vi "HandDetector.vi"(6 "Enum":T2, 8 "error in (no error)":errorcluster, 10 "Image":T1, 11 "session in":refnum<k35>) -> (0 "error out":errorcluster, 1 "Landmarkers coords":u32[][](array[numeric]), 2 "OutImage":T1, 3 "session out":refnum<k35>, 4 "HandExist?":bool)   [LabVIEW 2024]
uses:
  #VisionProcessingEnum.ctl
  <vilib>/vision/Image Controls.llb/IMAQ Image.ctl
  <vilib>/Python/Open Venv Python Session.vi
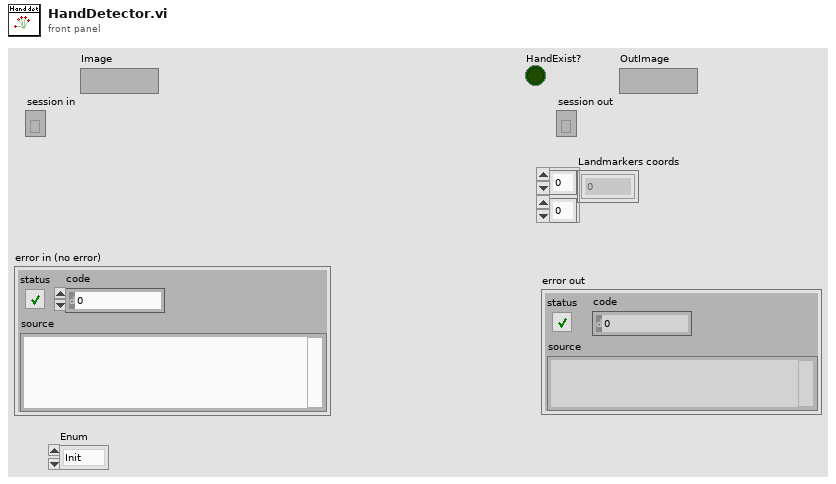
[diagram p1: front panel]
types:
  T1 = typedef "IMAQ Image.ctl" = refnum<image>
  T2 = typedef "#VisionProcessingEnum.ctl" = enum16{"Init", "Processing", "ProcessingVision", "Close"}
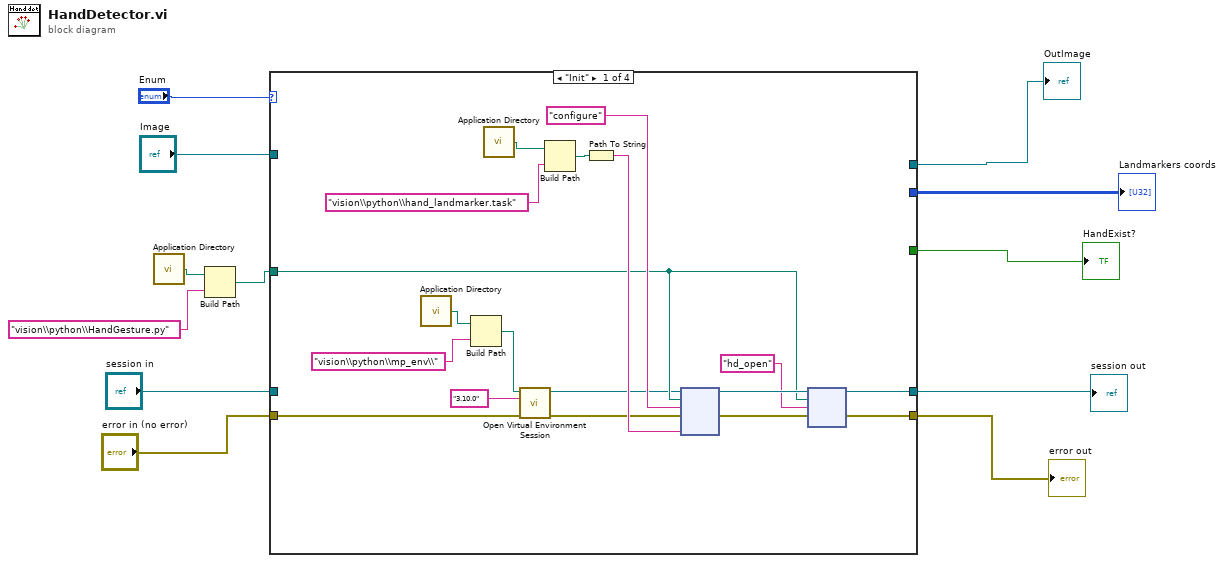
[diagram p0: block diagram]
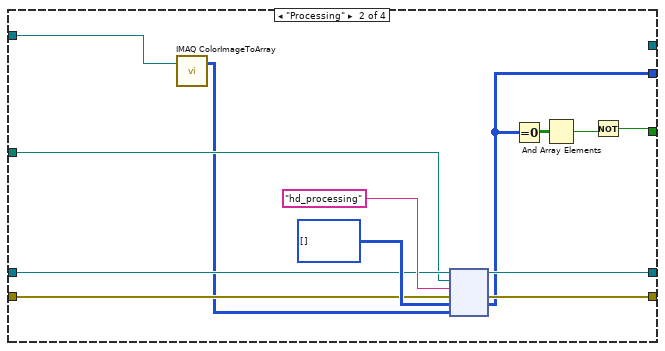
[diagram p2: hidden frame]
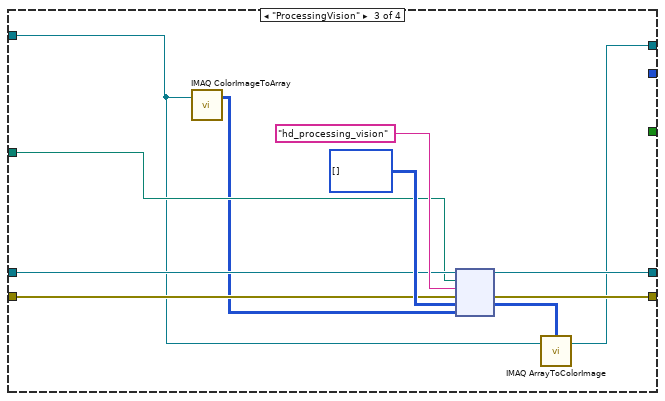
[diagram p3: hidden frame]
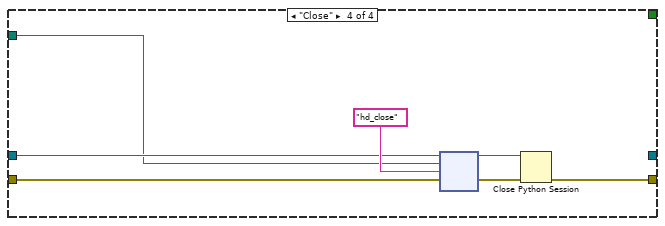
[diagram p4: hidden frame]
diagram:
  n1 = call <vilib>:"Application Directory.vi"() -> ("Application Directory"=w1:path)
  n2 = Build Path(base path=w1, name or relative path="vision\\python\\HandGesture.py" ("function name")) -> (appended path=w6:path)
  n3 = case shown="\"Init\"" "Enum" {
    tunnel: [w23 w40 w52 _] -> w9
    tunnel: [w22 w41 w50 w58] -> w8
    tunnel: "error in (no error)" -> [w13 w38 w49 w57]
    tunnel: "session in" -> [_ w39 w51 w56]
    tunnel: [_ _ w46 _] -> w4
    tunnel: w6 -> [w21 w37 w48 w55]
    tunnel: "Image" -> [_ w35 w44 _]
    tunnel: [_ w34 _ _] -> w3
    tunnel: [_ w31 _ _] -> w2
    frame "Init" {
      n4 = call <vilib>:"Application Directory.vi"() -> ("Application Directory"=w18:path)
      n5 = Build Path(base path=w18, name or relative path="vision\\python\\mp_env\\" ("function name")) -> (appended path=w19:path)
      n6 = call <vilib>:"Application Directory.vi"() -> ("Application Directory"=w20:path)
      n7 = call-poly <vilib>:"Open Virtual Environment Session.vi"("error in (no error)"=w13, "Python version"="3.10.0", "Env path"=w19) -> ("error out"=w15:errorcluster, "session out"=w14:refnum<k35>)  [unwired: 7 in]
      n8 = Build Path(base path=w20, name or relative path="vision\\python\\hand_landmarker.task" ("function name")) -> (appended path=w27:path)
      n9 = Path To String(path=w27) -> (string=w28:string)
      n10 = node(w14, w21, "configure" ("function name"), w15, w28) -> (w29:refnum<k35>, w30:errorcluster)  [unwired: 3 in, 2 out]
      n11 = node(w29, w21, "hd_open" ("function name"), w30) -> (w23:refnum<k35>, w22:errorcluster)  [unwired: 2 in, 2 out]
    }
    frame "Processing" {
      n12 = call "IMAQ ColorImageToArray"("Image"=w35) -> ("Image Pixels (U32)"=w36:u32[][])  [unwired: 3 in, 2 out]
      n13 = node(w39, w37, "hd_processing" ("function name"), w38, u32[][] [], w36) -> (w40:refnum<k35>, w41:errorcluster, w34:u32[][])  [unwired: 1 in, 2 out]
      n14 = Equal To 0?(x=w34) -> (x = 0?=w33:bool[][])
      n15 = And Array Elements(Boolean array=w33) -> (logical AND=w32:bool)
      n16 = Not(x=w32) -> (.not. x?=w31:bool)
    }
    frame "ProcessingVision" {
      n17 = call "IMAQ ColorImageToArray"("Image"=w44) -> ("Image Pixels (U32)"=w47:u32[][])  [unwired: 3 in, 2 out]
      n18 = node(w51, w48, "hd_processing_vision" ("function name"), w49, u32[][] [], w47) -> (w52:refnum<k35>, w50:errorcluster, w45:u32[][])  [unwired: 1 in, 2 out]
      n19 = call "IMAQ ArrayToColorImage"("Image Pixels (U32)"=w45, "Image"=w44) -> ("Image Out"=w46:T1)  [unwired: 3 in, 1 out]
    }
    frame "Close" {
      n20 = node(w56, w55, "hd_close" ("function name"), w57) -> (w60:refnum<k35>, w59:errorcluster)  [unwired: 2 in, 2 out]
      n21 = Close Python Session(session in=w60, error in=w59) -> (11:w58:errorcluster)
    }
  }
  "session out" <- w9
  "error out" <- w8
  "Landmarkers coords" <- w3
  "OutImage" <- w4
  "HandExist?" <- w2
